vi "Unit Test 2.vi"() -> ()   [LabVIEW 2018]
uses:
  3446X.lvclass
  3446X.lvclass/3446X.ctl
panel:
  out "error out 4":errorcluster
  out "error out 3":errorcluster
  out "error out 2":errorcluster
  in  "Instr Resource":refnum<visa-resource-name>
  in  "OK Button":bool
  in  "stop":bool
  out "error out":errorcluster
  in  "error in (no error)":errorcluster
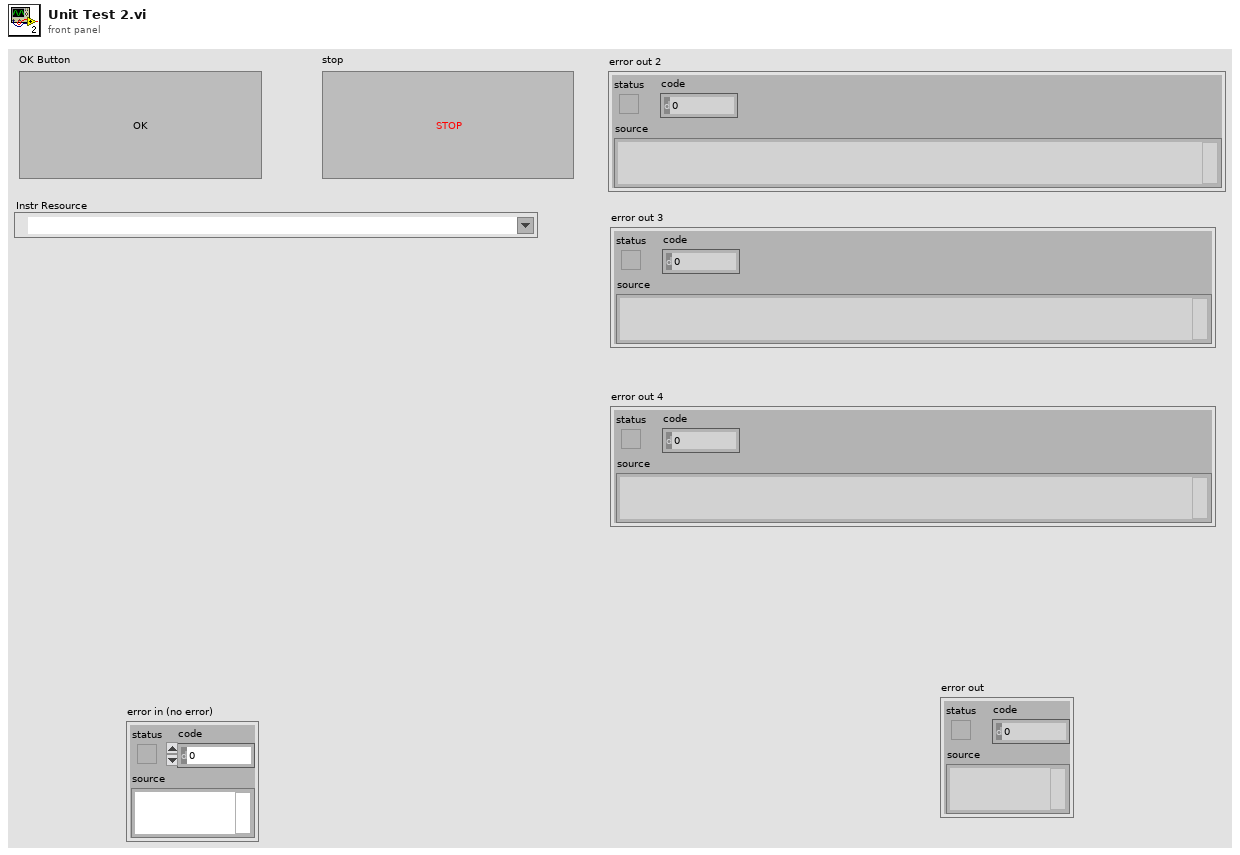
[diagram p1: front panel]
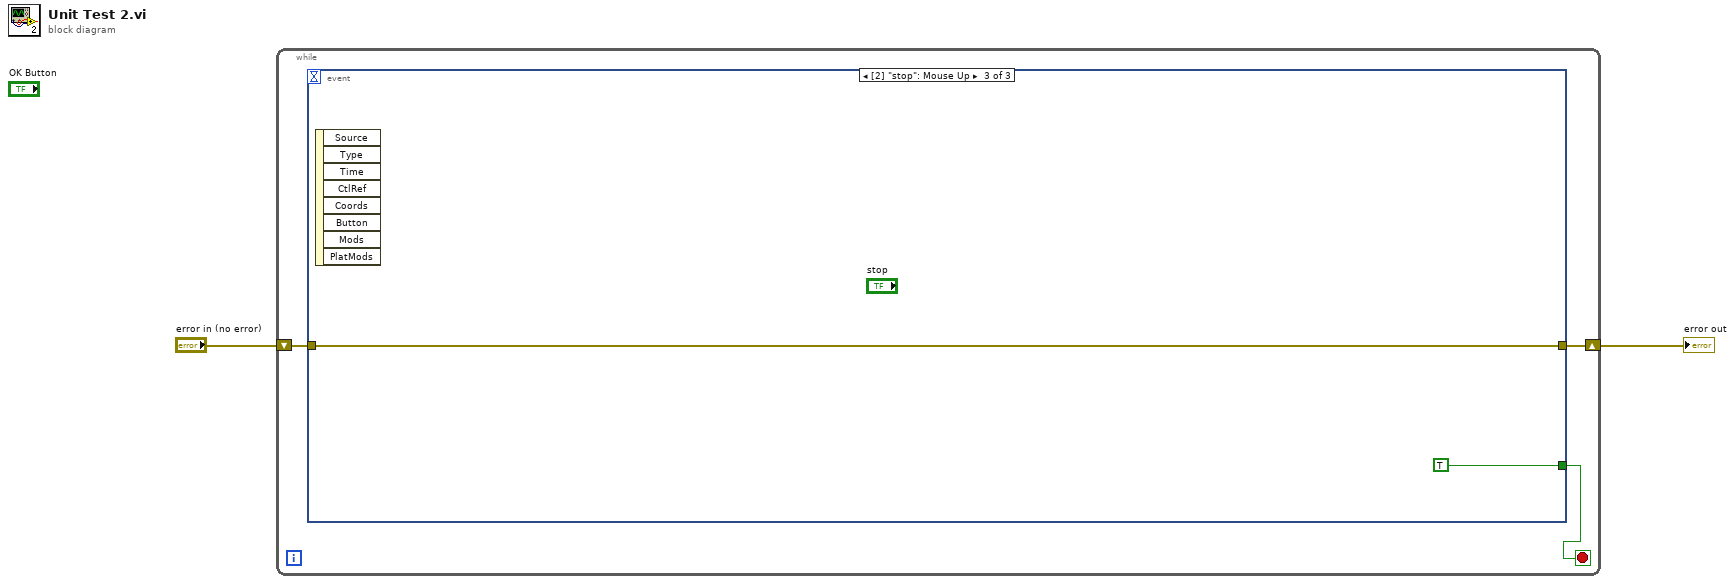
[diagram p0: block diagram]
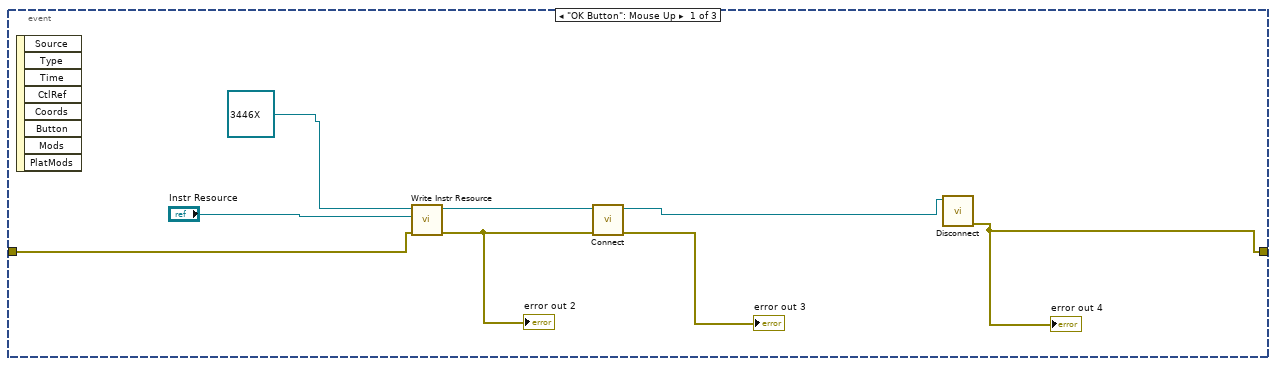
[diagram p2: hidden frame]
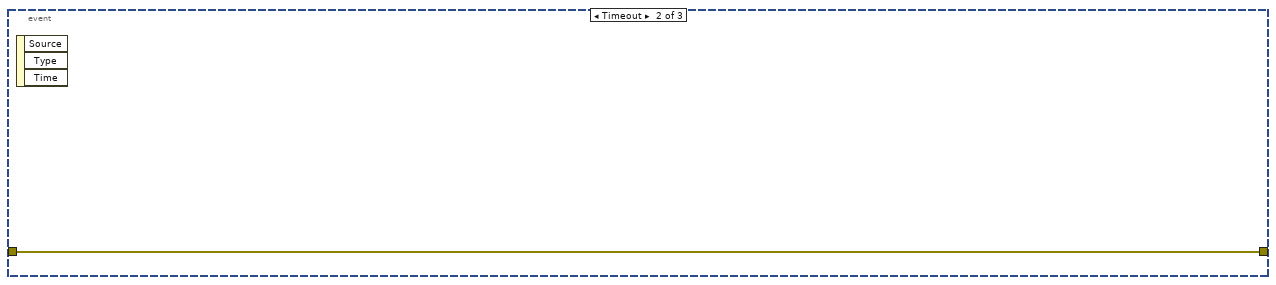
[diagram p3: hidden frame]
diagram:
  n1 = while {
    shift-right: [w4] -> w1
    shift-left: "error in (no error)" -> [w5]
    stop <- w3 stop-if-true
    n2 = event shown="[2] \"stop\": Mouse Up" {
      selector: _ -> [_ _ _]
      dyn-events: _ -> [_ _ _]
      timeout: _ -> [_ _ _]
      tunnel: w5 -> [w11 w14 w16]
      tunnel: [w6 w14 w16] -> w4
      tunnel: [_ _ TRUE] -> w3
      event "OK Button": Mouse Up {
        n3 = event-data() -> ()  [unwired: 1 in, 8 out]
        n4 = call "Write Instr Resource.vi"("error in (no error)"=w11, "Instr Resource"="Instr Resource", "3446X in"=refnum<class "3446X.lvclass"> refnum ("3446X.lvlib:3446X.lvclass")) -> ("error out"=w9:errorcluster, "3446X out"=w10:refnum<class "3446X.lvclass">)  [unwired: 7 in]
        "error out 2" <- w9
        n5 = call-dynamic "Connect.vi"("error in (no error)"=w9, "3446X in"=w10) -> ("error out"=→"error out 3":errorcluster, "3446X out"=w8:refnum<class "3446X.lvclass">)  [unwired: 8 in]
        n6 = call-dynamic "Disconnect.vi"("3446X in"=w8) -> ("error out"=w6:errorcluster)  [unwired: 9 in, 1 out]
        "error out 4" <- w6
      }
      event Timeout {
        n7 = event-data() -> ()  [unwired: 1 in, 3 out]
      }
      event "stop": Mouse Up {
        n8 = event-data() -> ()  [unwired: 1 in, 8 out]
      }
    }
  }
  "error out" <- w1
